vi "Shooter Lookup Table.vi"(9 "Sonar Value":dbl, 11 "Final(t) Slop(f)":bool) -> (1 "Hood":dbl, 3 "RPM":dbl)   [LabVIEW 2017, in "Shooter.lvlib"]
uses:
  Shooter.lvlib
  TypeDefs/ENUM_Shooter column Lookup table.ctl
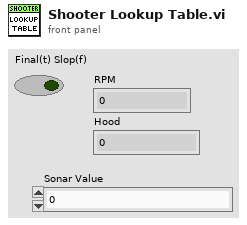
[diagram p1: front panel]
types:
  T1 = typedef "ENUM_Shooter column Lookup table.ctl" = enum16{"Distance Sonar Final", "Distance Sonar Slop", "RPM", "Hood Angle"}
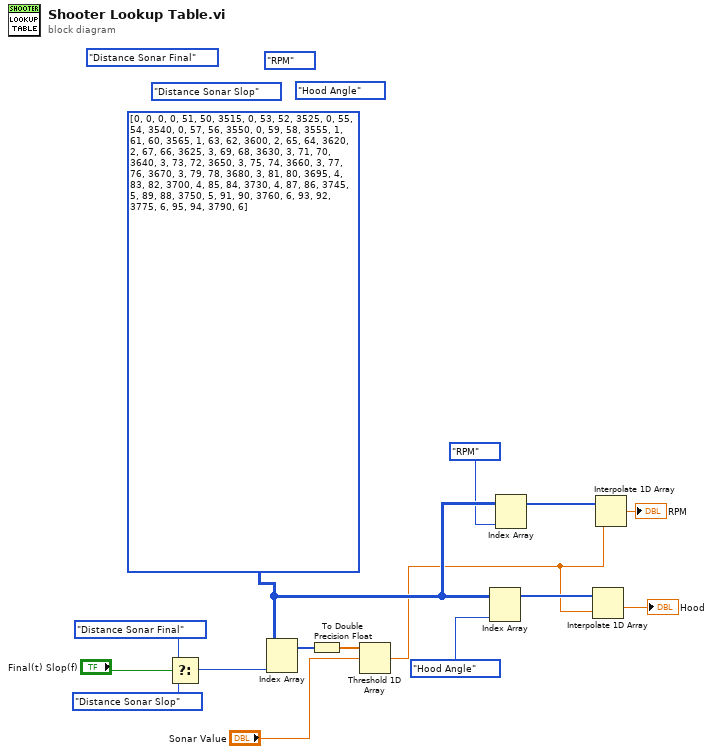
[diagram p0: block diagram]
diagram:
  (unwired) ENUM_Shooter_column_Lookup_table."Hood Angle" ("Shooter Lookup columns 2")
  (unwired) ENUM_Shooter_column_Lookup_table."RPM" ("Shooter Lookup columns 2")
  (unwired) ENUM_Shooter_column_Lookup_table."Distance Sonar Slop" ("Shooter Lookup columns 2")
  (unwired) ENUM_Shooter_column_Lookup_table."Distance Sonar Final" ("Shooter Lookup columns 2")
  w10 = i32[][] [[0, 0, 0, 0], [51, 50, 3515, 0], [53, 52, 3525, 0], [55, 54, 3540, 0], [57, 56, 3550, 0], [59, 58, 3555, 1], [61, 60, 3565, 1], [63, 62, 3600, 2], [65, 64, 3620, 2], [67, 66, 3625, 3], [69, 68, 3630, 3], [71, 70, 3640, 3], [73, 72, 3650, 3], [75, 74, 3660, 3], [77, 76, 3670, 3], [79, 78, 3680, 3], [81, 80, 3695, 4], [83, 82, 3700, 4], [85, 84, 3730, 4], [87, 86, 3745, 5], [89, 88, 3750, 5], [91, 90, 3760, 6], [93, 92, 3775, 6], [95, 94, 3790, 6]] ("array")
  n1 = Select(t=ENUM_Shooter_column_Lookup_table."Distance Sonar Final" ("Shooter Lookup columns"), s="Final(t) Slop(f)", f=ENUM_Shooter_column_Lookup_table."Distance Sonar Slop" ("Shooter Lookup columns")) -> (s? t:f=w12:T1)
  n2 = Index Array(array=w10, index (col)=w12) -> (element=w11:i32[])  [unwired: 1 in]
  n3 = To Double Precision Float(number=w11) -> (double precision float=w2:dbl[])
  n4 = Threshold 1D Array(2:"Sonar Value", 3:w2) -> (0:w5:dbl)  [unwired: 1 in]
  n5 = Index Array(array=w10, index (col)=ENUM_Shooter_column_Lookup_table."Hood Angle" ("Shooter Lookup columns")) -> (element=w6:i32[])  [unwired: 1 in]
  n6 = Index Array(array=w10, index (col)=ENUM_Shooter_column_Lookup_table."RPM" ("Shooter Lookup columns")) -> (element=w7:i32[])  [unwired: 1 in]
  n7 = Interpolate 1D Array(1:w5, 2:w6) -> (0:→"Hood":dbl)
  n8 = Interpolate 1D Array(1:w5, 2:w7) -> (0:→"RPM":dbl)
